vi "VI-Wire Reg Events Terminals.vi"(0 "VI in":refnum<vi>, 2 "Components":T1, 9 "Num refs":i32, 11 "error in (no error)":errorcluster) -> (4 "VI out":refnum<vi>, 15 "error out":errorcluster)   [LabVIEW 2015]
uses:
  VI-Reg Event Components.ctl
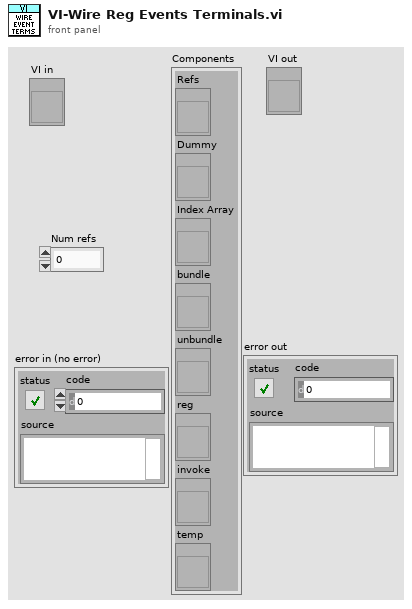
[diagram p1: front panel]
types:
  T1 = typedef "VI-Reg Event Components.ctl" = cluster{"Refs":refnum<vi>, "Dummy":refnum<vi>, "Index Array":refnum<vi>, "bundle":refnum<vi>, "unbundle":refnum<vi>, "reg":refnum<vi>, "invoke":refnum<vi>, "temp":refnum<vi>}
  T2 = typedef "LVPositionTypeDef.ctl" = cluster{"Left":i32, "Top":i32}
  T3 = typedef "LVRectTypeDef.ctl" = cluster{"Left":i16, "Top":i16, "Right":i16, "Bottom":i16}
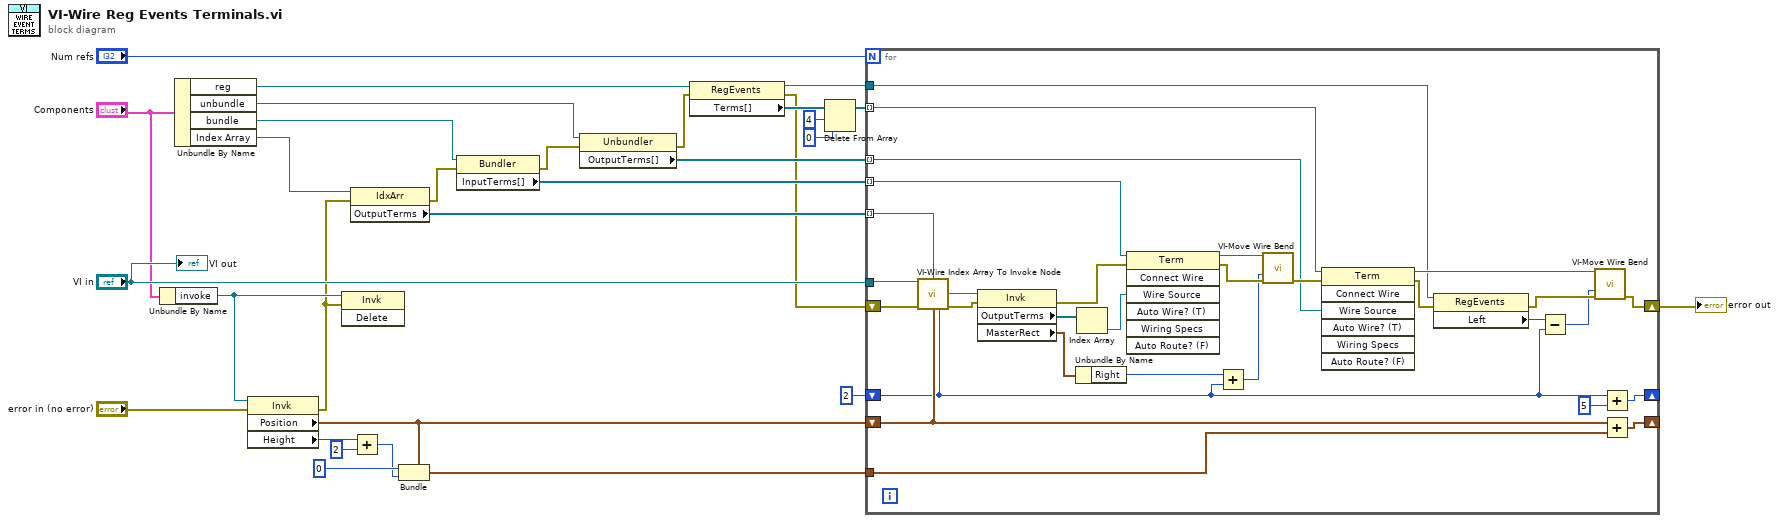
[diagram p0: block diagram]
diagram:
  n1 = Unbundle By Name("Components") -> ("invoke"=w2:refnum<vi>)
  n2 = Unbundle By Name("Components") -> ("reg"=w12:refnum<vi>, "unbundle"=w14:refnum<vi>, "bundle"=w16:refnum<vi>, "Index Array"=w19:refnum<vi>)
  n3 = property class="Invk"(reference=w2, error in="error in (no error)") -> (error out=w1:errorcluster, "Position"=w21:T2, "Height"=w27:u32)  [unwired: 1 out]
  n4 = invoke class="Invk" method="Delete"(reference=w2, error in=w1) -> ()  [unwired: 1 in, 3 out]
  n5 = property class="IdxArr"(reference=w19, error in=w1) -> (error out=w17:errorcluster, "OutputTerms"=w18:refnum<vi>[])  [unwired: 1 out]
  n6 = Add(x=w27, y=u32 2) -> (x+y=w24:u32)
  n7 = Bundle(cluster=w21, "Left"=0, "Top"=w24) -> (w22:T2)
  n8 = property class="Bundler"(reference=w16, error in=w17) -> (error out=w15:errorcluster, "InputTerms[]"=w9:refnum<vi>[])  [unwired: 1 out]
  n9 = property class="Unbundler"(reference=w14, error in=w15) -> (error out=w13:errorcluster, "OutputTerms[]"=w10:refnum<vi>[])  [unwired: 1 out]
  n10 = property class="RegEvents"(reference=w12, error in=w13) -> (reference out=w6:refnum<vi>, error out=w8:errorcluster, "Terms[]"=w11:refnum<vi>[])
  n11 = Delete From Array(array=w11, length=4, index=0) -> (array with subset deleted=w5:refnum<vi>[])  [unwired: 1 out]
  n12 = for {
    N: "Num refs" -> [_]
    tunnel: "VI in" -> [w56]
    shift-right: [w32] -> w28
    shift-left: w8 -> [w58]
    tunnel: w22 -> [w59]
    shift-right: [w60] -> _
    shift-left: w21 -> [w57]
    tunnel: w18 -> [w51] mode=indexing
    tunnel: w5 -> [w38] mode=indexing
    tunnel: w10 -> [w40] mode=indexing
    tunnel: w9 -> [w43] mode=indexing
    shift-right: [w55] -> _
    shift-left: 2 -> [w34]
    tunnel: w6 -> [w37]
    n13 = call "VI-Wire Index Array To Invoke Node.vi"("VI in"=w56, "Index Array ref"=w51, "error in (no error)"=w58, "Position"=w57, "Xbend"=w34) -> ("invoke node ref"=w52:refnum<vi>, "error out"=w53:errorcluster)  [unwired: 9 in]
    n14 = property class="Invk"(reference=w52, error in=w53) -> (error out=w49:errorcluster, "OutputTerms"=w50:refnum<vi>[], "MasterRect"=w44:T3)  [unwired: 1 out]
    n15 = Unbundle By Name(w44) -> ("Right"=w46:i16)
    n16 = Index Array(array=w50) -> (element=w42:refnum<vi>)  [unwired: 1 in]
    n17 = invoke class="Term" method="Connect Wire"(reference=w43, error in=w49, "Wire Source"=w42) -> (reference out=w48:refnum<vi>, error out=w47:errorcluster)  [unwired: 4 in, 5 out]
    n18 = Add(x=w46, y=w34) -> (x+y=w45:i32)
    n19 = call "VI-Move Wire Bend.vi"("Terminal in"=w48, "Horizontal"=w45, "error in (no error)"=w47) -> ("error out"=w41:errorcluster)  [unwired: 12 in]
    n20 = invoke class="Term" method="Connect Wire"(reference=w38, error in=w41, "Wire Source"=w40) -> (reference out=w39:refnum<vi>, error out=w36:errorcluster)  [unwired: 4 in, 5 out]
    n21 = property class="RegEvents"(reference=w37, error in=w36) -> (error out=w35:errorcluster, "Left"=w31:i32)  [unwired: 1 out]
    n22 = Subtract(x=w31, y=w34) -> (x-y=w33:i32)
    n23 = call "VI-Move Wire Bend.vi"("Terminal in"=w39, "Horizontal"=w33, "error in (no error)"=w35) -> ("error out"=w32:errorcluster)  [unwired: 12 in]
    n24 = Add(x=w34, y=5) -> (x+y=w55:i32)
    n25 = Add(x=w57, y=w59) -> (x+y=w60:T2)
  }
  "error out" <- w28
  "VI out" <- "VI in"
